vi "QUERY_TELEM.vi"() -> ()   [LabVIEW 2023, in "Clover_Cell.lvlib"]
uses:
  Clover_Cell.lvlib
panel:
  in  "TRXmode":u16(ring)=1 items=["QUERY_TELEM_2 (V)"=2, "QUERY_TELEM_1 (H)"=1]
  in  "TCPIPin":T1={"address"="192.168.100.111", "remote port or service name"=5025, "timeout ms (60000)"=10000}
  out "L2":T2(array[cluster])
  out "size(s)":i32
  # "AiP_1 : 0\nAiP_2 : 1\nAiP_3 : 2\nAiP_4 : 3\nAiP_5 : 4\nAiP_6 : 5\nAiP_7 : 6\nAiP_8 : 7"
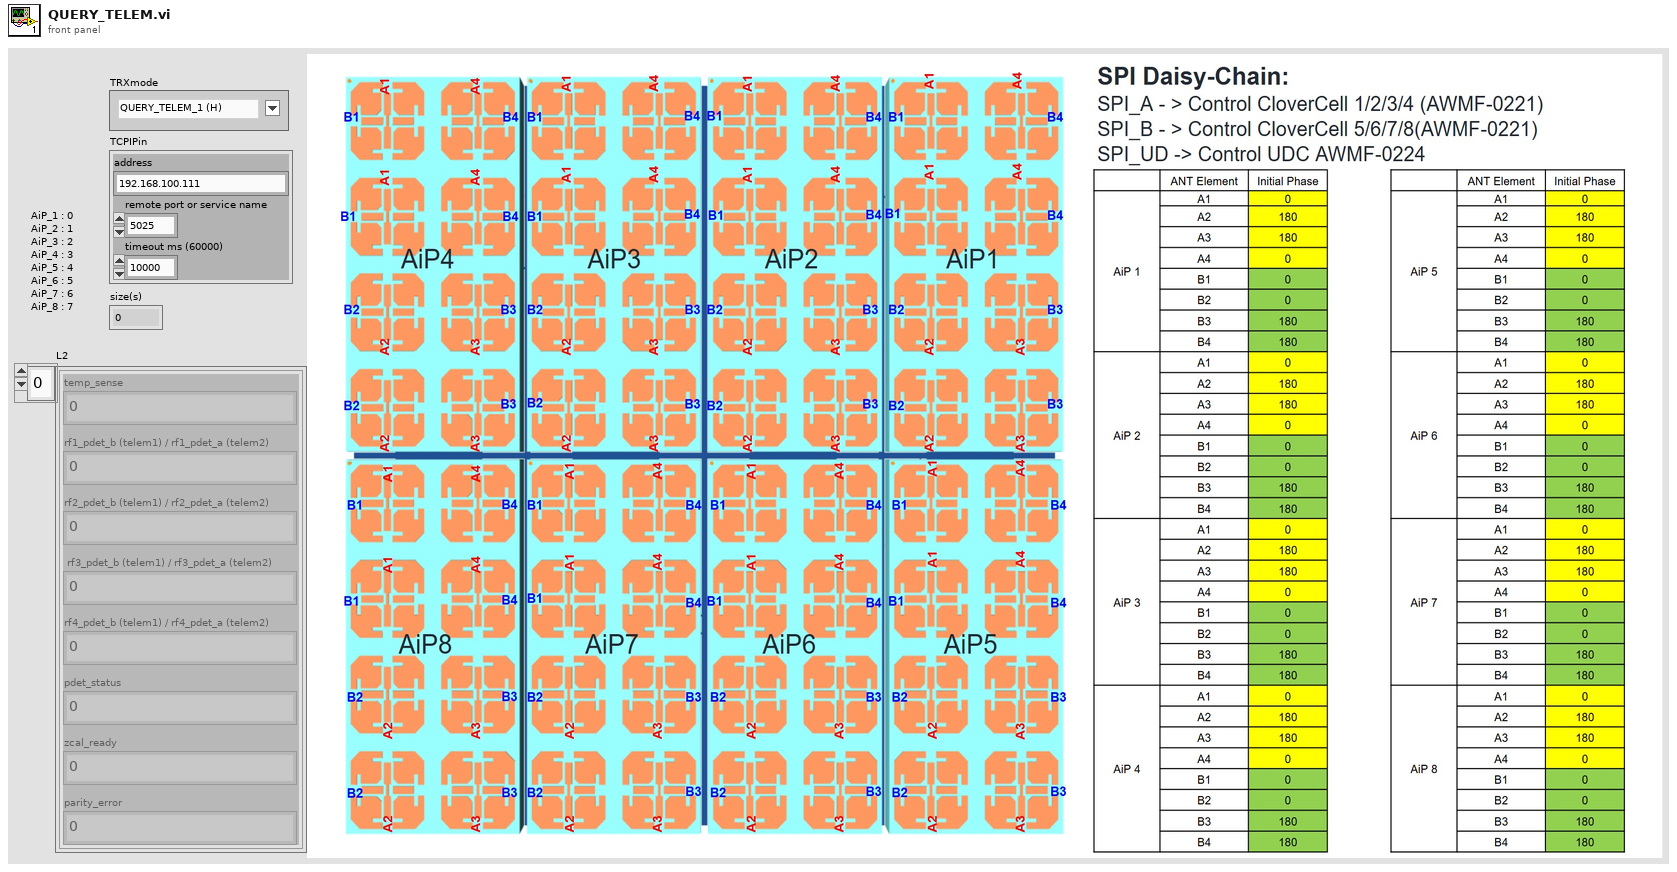
[diagram p1: front panel]
types:
  T1 = cluster{"address":string, "remote port or service name":u16, "timeout ms (60000)":i32}
  T2 = cluster{"temp_sense":i32, "rf1_pdet_b (telem1) / rf1_pdet_a (telem2)":i32, "rf2_pdet_b (telem1) / rf2_pdet_a (telem2)":i32, " rf3_pdet_b (telem1) / rf3_pdet_a (telem2)":i32, "rf4_pdet_b (telem1) / rf4_pdet_a (telem2)":i32, "pdet_status":i32, "zcal_ready":i32, "parity_error":i32}[]
  T3 = cluster{"temp_sense":i32, "rf1_pdet_b (telem1) / rf1_pdet_a (telem2)":i32, "rf2_pdet_b (telem1) / rf2_pdet_a (telem2)":i32, " rf3_pdet_b (telem1) / rf3_pdet_a (telem2)":i32, "rf4_pdet_b (telem1) / rf4_pdet_a (telem2)":i32, "pdet_status":i32, "zcal_ready":i32, "parity_error":i32}
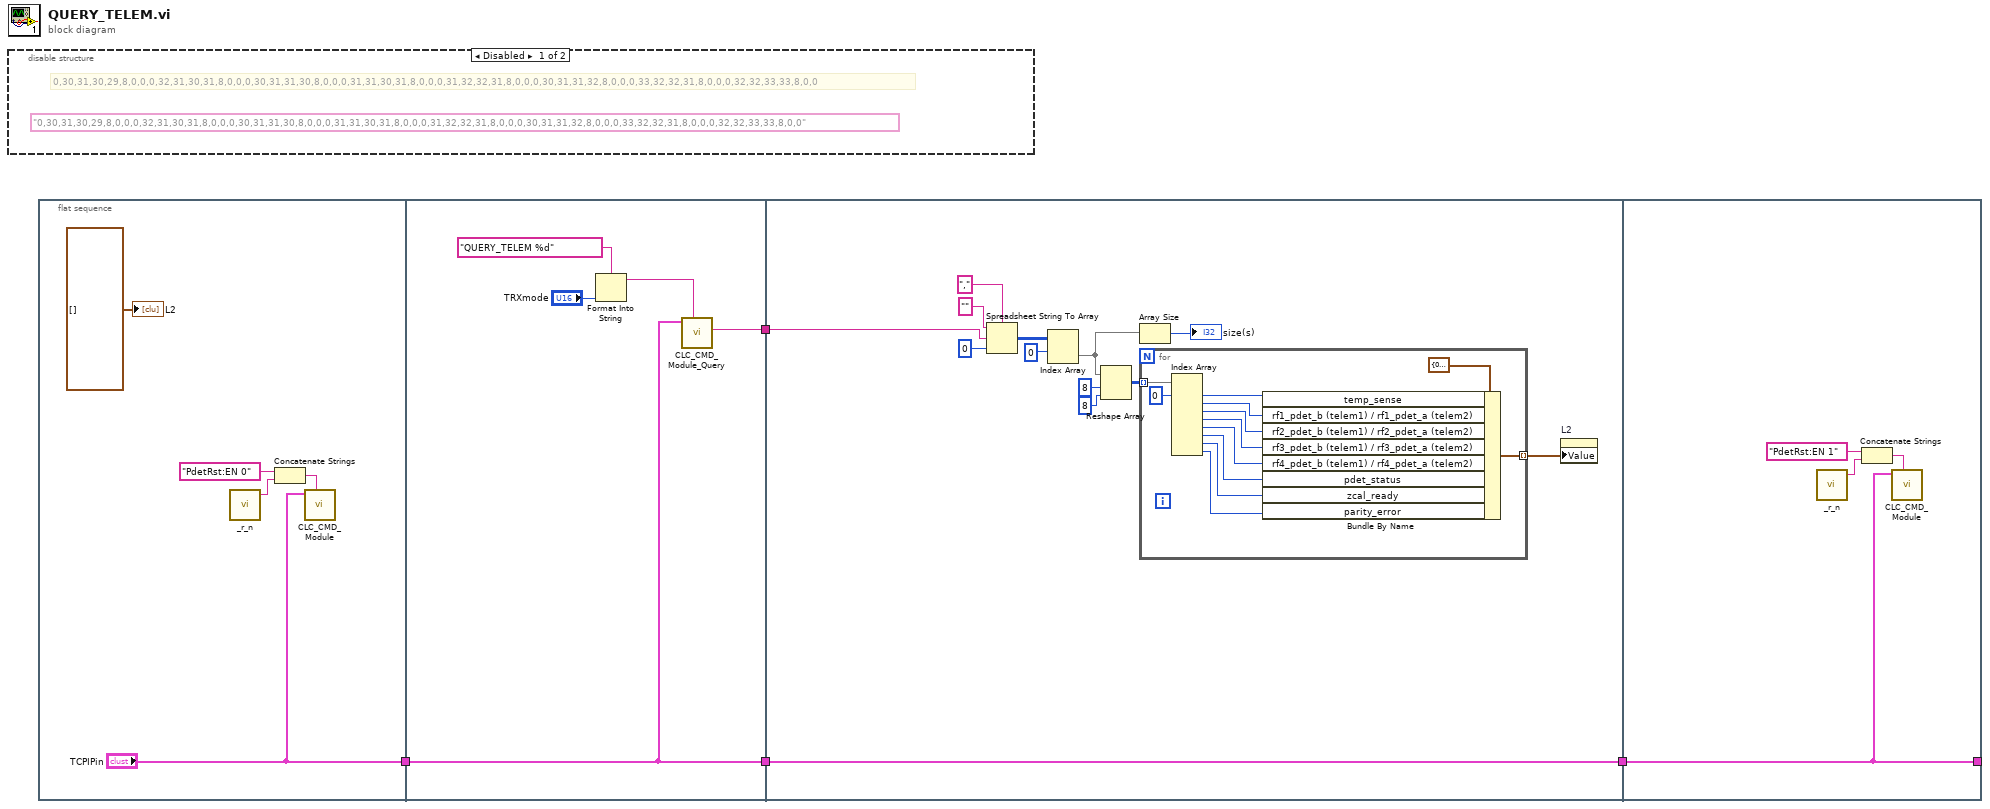
[diagram p0: block diagram]
diagram:
  n1 = disable-structure shown="Disabled" {
    frame Disabled {
      (unwired) "0,30,31,30,29,8,0,0,0,32,31,30,31,8,0,0,0,30,31,31,30,8,0,0,0,31,31,30,31,8,0,0,0,31,32,32,31,8,0,0,0,30,31,31,32,8,0,0,0,33,32,32,31,8,0,0,0,32,32,33,33,8,0,0"
      # "0,30,31,30,29,8,0,0,0,32,31,30,31,8,0,0,0,30,31,31,30,8,0,0,0,31,31,30,31,8,0,0,0,31,32,32,31,8,0,0,0,30,31,31,32,8,0,0,0,33,32,32,31,8,0,0,0,32,32,33,33,8,0,0"
    }
    frame Enabled {
    }
  }
  n2 = flat-sequence {
    tunnel: ["TCPIPin"] -> w2
    tunnel: [w14] -> w4
    tunnel: [w10] -> w3
    tunnel: w2 -> [w10]
    tunnel: w4 -> [w25]
    tunnel: w3 -> [w15]
    tunnel: [w15] -> w1
    tunnel: [w40] -> _
    tunnel: w1 -> [w40]
    frame #0 {
      n3 = call "_r_n.vi"() -> ("command"=w7:string)  [unwired: 5 in]
      n4 = Concatenate Strings("PdetRst:EN 0" ("CMD in"), w7) -> (w6:string)
      n5 = call "CLC_CMD_Module.vi"("CMD in"=w6, "TCPIPin"="TCPIPin") -> ()  [unwired: 6 in, 4 out]
      "L2" <- T2 [] ("L2")
    }
    frame #1 {
      n6 = Format Into String(format string="QUERY_TELEM %d" ("data in"), "TRXmode") -> (resulting string=w11:string)  [unwired: 2 in, 1 out]
      n7 = call "CLC_CMD_Module_Query.vi"("CMD in"=w11, "TCPIPin"=w10) -> ("data out"=w14:string)  [unwired: 7 in, 2 out]
    }
    frame #2 {
      n8 = Spreadsheet String To Array(delimiter (Tab)=",", format string="", spreadsheet string=w25, array type (2D Dbl)=0) -> (array=w21:i32[][])
      n9 = Index Array(array=w21, index (row)=0 ("disabled index (col)")) -> (element=w19:i32[])  [unwired: 1 in]
      n10 = Reshape Array(w19, 8 ("dimension size"), 8 ("dimension size")) -> (w17:i32[][])
      n11 = Array Size(array=w19) -> (size(s)=→"size(s)":i32)
      n12 = for {
        tunnel: w17 -> [w39] mode=indexing
        tunnel: [w28] -> w16 mode=indexing
        n13 = Index Array(array=w39, index #1=0 ("index")) -> (element #1=w37:i32, element #2=w36:i32, element #3=w34:i32, element #4=w33:i32, element #5=w32:i32, element #6=w31:i32, element #7=w30:i32, element #8=w29:i32)  [unwired: 7 in]
        n14 = Bundle By Name(cluster=T3 {"temp_sense"=0, "rf1_pdet_b (telem1) / rf1_pdet_a (telem2)"=0, "rf2_pdet_b (telem1) / rf2_pdet_a (telem2)"=0, " rf3_pdet_b (telem1) / rf3_pdet_a (telem2)"=0, "rf4_pdet_b (telem1) / rf4_pdet_a (telem2)"=0, "pdet_status"=0, "zcal_ready"=0, "parity_error"=0} ("L2 Information"), "temp_sense"=w37, "rf1_pdet_b (telem1) / rf1_pdet_a (telem2)"=w36, "rf2_pdet_b (telem1) / rf2_pdet_a (telem2)"=w34, "rf3_pdet_b (telem1) / rf3_pdet_a (telem2)"=w33, "rf4_pdet_b (telem1) / rf4_pdet_a (telem2)"=w32, "pdet_status"=w31, "zcal_ready"=w30, "parity_error"=w29) -> (w28:T3)
      }
      n15 = property on="L2" class="Arr (strict)"("Value"=w16) -> ()  [unwired: 2 in, 2 out]
    }
    frame #3 {
      n16 = call "_r_n.vi"() -> ("command"=w42:string)  [unwired: 5 in]
      n17 = Concatenate Strings("PdetRst:EN 1" ("CMD in"), w42) -> (w43:string)
      n18 = call "CLC_CMD_Module.vi"("CMD in"=w43, "TCPIPin"=w40) -> ()  [unwired: 6 in, 4 out]
    }
  }
